vi "String_to_XYZ_Pos.vi"(0 "Input string":string, 1 "Position label":string) -> (2 "X":dbl format="%.2f", 3 "Y":dbl format="%.2f", 4 "Z":dbl format="%.2f")   [LabVIEW 2010]
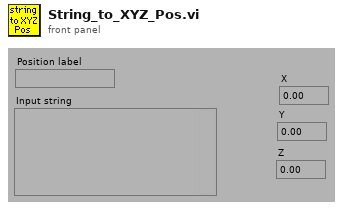
[diagram p1: front panel]
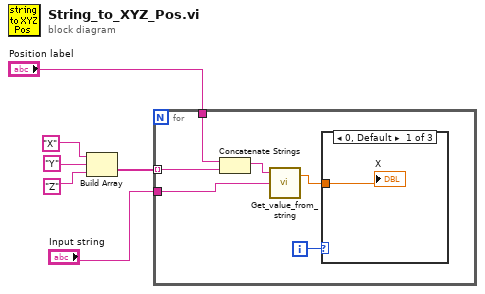
[diagram p0: block diagram]
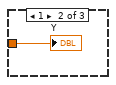
[diagram p2: hidden frame]
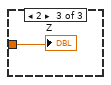
[diagram p3: hidden frame]
diagram:
  n1 = Build Array("X", "Y", "Z") -> (w6:string[])
  n2 = for {
    tunnel: "Position label" -> [w7]
    tunnel: w6 -> [w12] mode=indexing
    tunnel: "Input string" -> [w10]
    i -> [w9]
    n3 = Concatenate Strings(w7, w12) -> (w11:string)
    n4 = call "Get_value_from_string.vi"("Input string"=w10, "Variable name"=w11) -> ("Value"=w8:dbl)  [unwired: 1 in, 1 out]
    n5 = case shown="0, Default" w9 {
      tunnel: w8 -> [w13 w14 w15]
      frame 0, Default {
        "X" <- w13
      }
      frame 1 {
        "Y" <- w14
      }
      frame 2 {
        "Z" <- w15
      }
    }
  }
